vi "set_process_layer_parameter.vi"(6 "Layer number":u8=1 min=1 max=200 step=1, 7 "Parameter value":variant, 8 "error in (no error)":errorcluster, 9 "Process number":u8=1 min=1 max=50 step=1, 10 "Process layer parameter":T1 items=["Material", "Final Thick (kA)", "Thick Limit (kA)", "Crucible", "CoDep", "Ratio Cntrl (%)"], 11 "VISA resource name":refnum<visa-resource-name>) -> (0 "error out":errorcluster, 3 "VISA resource name out":refnum<visa-resource-name>)   [LabVIEW 2018]
doc: "Set the density of a material."
uses:
  Low Level/process_layer_parameter_ring.ctl
panel:
  out "formatted response":string
  out "command packet":string
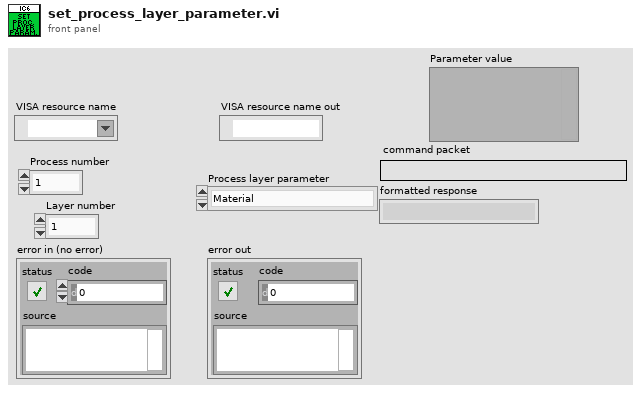
[diagram p1: front panel]
types:
  T1 = typedef "process_layer_parameter_ring.ctl" = u16
  T2 = enum16{"Source", "General", "Input name", "Process name", "Logic", "Material", "Material name", "Output name", "Process", "Sensor", "Output type", "User message", "Layer", ""}
  T3 = enum16{"Hello", "Query", "Remote action", "Status", "Update"}
  T4 = cluster{"Process number":u8, "Layer number":u8, "Parameter value":variant}
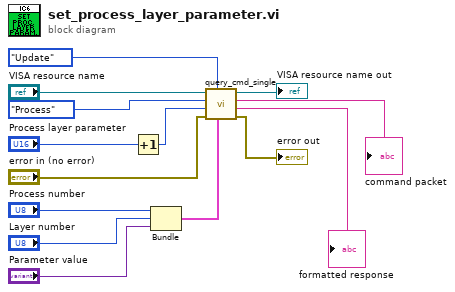
[diagram p0: block diagram]
diagram:
  n1 = Increment(x="Process layer parameter") -> (x+1=w7:T1)
  n2 = Bundle("Process number"="Process number", "Layer number"="Layer number", "Parameter value"="Parameter value") -> (w4:T4)  [unwired: 1 in]
  n3 = call "query_cmd_single.vi"("Parameter"=w4, "Command group"=T3."Update", "error in (no error)"="error in (no error)", "Command ID"=w7, "Command subgroup"=T2."Process", "VISA resource name"="VISA resource name") -> ("error out"=→"error out":errorcluster, "formatted response"=→"formatted response":string, "command packet"=→"command packet":string, "VISA resource name out"=→"VISA resource name out":refnum<visa-resource-name>)  [unwired: 1 in, 1 out]
